vi "Combine Authenticate Parameters.vi"(8 "error in (no error)":errorcluster, 11 "OAuth Credentials":T1={"Consumer Key"="", "Signature Method"=enum."HMAC-SHA1", "Token"="", "Version"="1.0", "Token Secret"="", "Consumer Secret"=""}) -> (0 "error out":errorcluster, 3 "Authentication Parameters":T3[](array[typedef]))   [LabVIEW 2011, in "i3-oauth.lvlib"]
doc: "Use this template to build a VI to use as a subVI."
uses:
  i3-oauth.lvlib
  Controls/key-value-pairs.ctl
  Controls/OAuth Credentials.ctl
  Controls/Signature Method.ctl
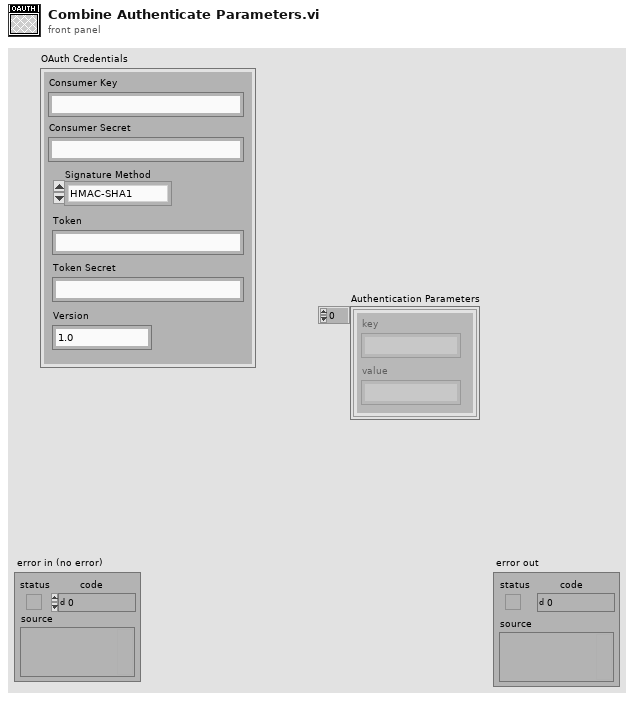
[diagram p1: front panel]
types:
  T1 = typedef "i3-oauth.lvlib/OAuth Credentials.ctl" = cluster{"Consumer Key":string, "Signature Method":T2, "Token":string, "Version":string, "Token Secret":string, "Consumer Secret":string}
  T2 = typedef "i3-oauth.lvlib/Signature Method.ctl" = enum16{"HMAC-MD5", "HMAC-SHA1", "HMAC-SHA224", "HMAC-SHA256", "HMAC-SHA384", "HMAC-SHA512"}
  T3 = typedef "i3-oauth.lvlib/key-value-pairs.ctl" = cluster{"key":string, "value":string}
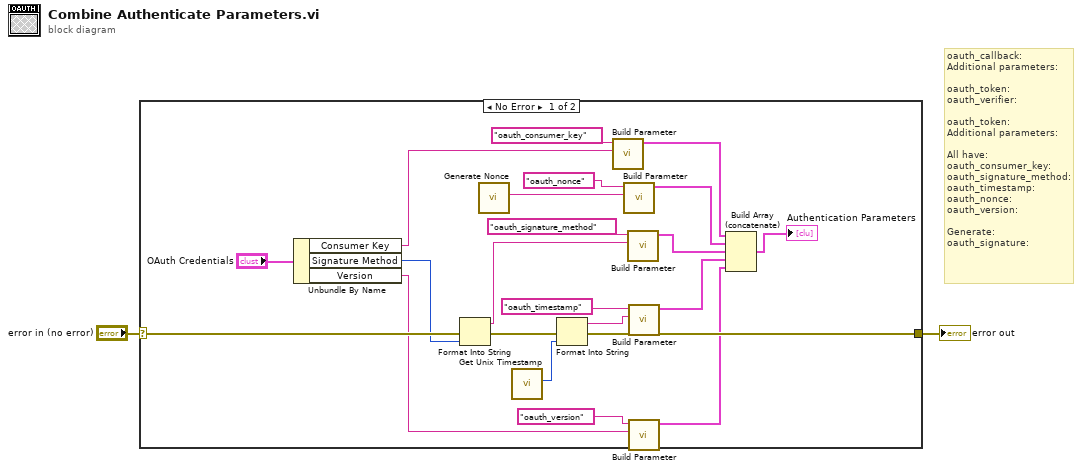
[diagram p0: block diagram]
diagram:
  # "oauth_callback:\nAdditional parameters:\n\noauth_token:\noauth_verifier:\n\noauth_token:\nAdditional parameters:\n\nAll have:\noauth_consumer_key:\noauth_signature_method:\noauth_timestamp:\noauth_nonce:\noauth_version:\n\nGenerate:\noauth_signature:"
  n1 = case shown="No Error" "error in (no error)" {
    selector: "error in (no error)" -> [w23 w25]
    tunnel: [w24 w25] -> w1
    frame No Error {
      n2 = Unbundle By Name("OAuth Credentials") -> ("Consumer Key"=w19:string, "Signature Method"=w21:T2, "Version"=w12:string)
      n3 = Format Into String(error in=w23, w21) -> (resulting string=w16:string, error out=w5:errorcluster)  [unwired: 2 in]
      n4 = call "Generate Nonce.vi"() -> ("nonce"=w3:string)  [unwired: 11 in]
      n5 = call "Get Unix Timestamp.vi"() -> ("Unix Timestamp"=w4:u64)  [unwired: 11 in]
      n6 = Format Into String(error in=w5, w4) -> (resulting string=w14:string, error out=w24:errorcluster)  [unwired: 2 in]
      n7 = call "Build Parameter.vi"("Value"=w19, "Key"="oauth_consumer_key" ("key")) -> ("Parameter Array"=w11:T3[])  [unwired: 9 in]
      n8 = call "Build Parameter.vi"("Value"=w3, "Key"="oauth_nonce" ("key")) -> ("Parameter Array"=w10:T3[])  [unwired: 9 in]
      n9 = call "Build Parameter.vi"("Value"=w16, "Key"="oauth_signature_method" ("key")) -> ("Parameter Array"=w9:T3[])  [unwired: 9 in]
      n10 = call "Build Parameter.vi"("Value"=w14, "Key"="oauth_timestamp" ("key")) -> ("Parameter Array"=w8:T3[])  [unwired: 9 in]
      n11 = call "Build Parameter.vi"("Value"=w12, "Key"="oauth_version" ("key")) -> ("Parameter Array"=w7:T3[])  [unwired: 9 in]
      n12 = Build Array (concatenate)(w11, w10, w9, w8, w7) -> (→"Authentication Parameters":T3[])
    }
    frame Error {
    }
  }
  "error out" <- w1
